vi "GetCOMPortold.vi"(8 "error in (no error)":errorcluster caption="错误输入（无错误）") -> (0 "error out":errorcluster caption="错误输出", 2 "COMPort":refnum<visa-resource-name>[](array[refnum]))   [LabVIEW 2013]
uses:
  <vilib>/nisyscfg/Filter Mode.ctl
  <vilib>/nisyscfg/Close (System).vi
  <vilib>/nisyscfg/nisyscfg.lvlib
  <resource>/objmgr/nisysapi.rc
panel:
  out "数组":string[](array[string])
  out "Alias":string[](array[string])
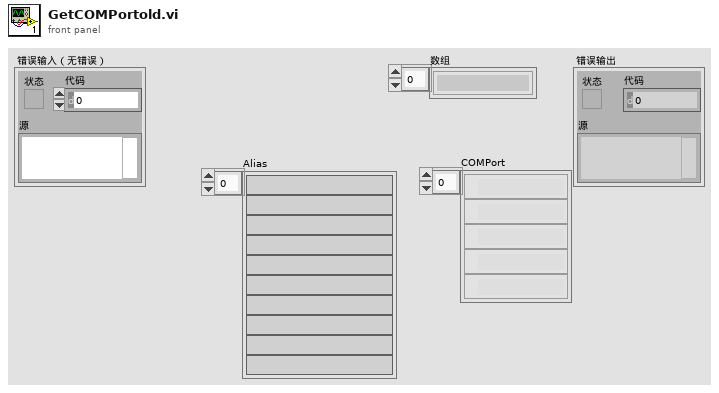
[diagram p1: front panel]
types:
  T1 = typedef "nisyscfg.lvlib/Filter Mode.ctl" = i32
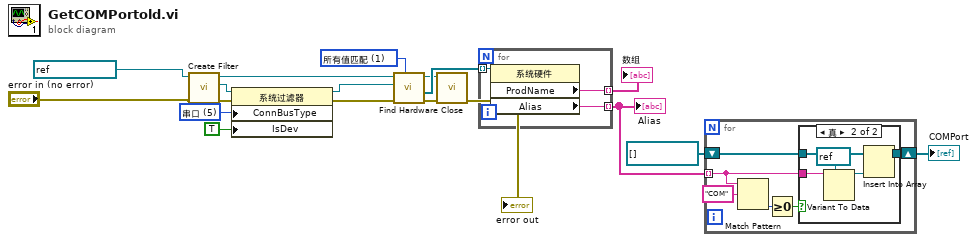
[diagram p0: block diagram]
diagram:
  w14 = u32 5 items=["内置/系统", "PXI/PCI", "USB", "GPIB", "VXI", "串口", "TCP/IP", "cRIO", "SCXI", "cDAQ", "SwitchBlock", "SCC", "FireWire", "FlexAdapter", "CAN"] ("设备与机箱:提供总线类型")
  w17 = T1 1 items=["所有值匹配"=1, "任意值匹配"=2, "值不匹配"=3, "所有属性存在"=4] ("Filter Mode (all values match)")
  n1 = call <vilib>:"Create Filter.vi"("error in (no error)"="error in (no error)", "Session in"=refnum<k21> "localhost") -> ("error out"=w16:errorcluster, "Filter out"=w10:refnum<k20>, "Session out"=w12:refnum<k21>)  [unwired: 7 in]
  n2 = property class="系统过滤器"(reference=w10, error in=w16, "ConnBusType"=w14, "IsDev"=TRUE ("属于设备")) -> (reference out=w9:refnum<k20>, error out=w11:errorcluster)
  n3 = call <vilib>:"Find Hardware.vi"("Filter Mode (all values match)"=w17, "error in (no error)"=w11, "Filter in"=w9, "Session in"=w12) -> ("error out"=w13:errorcluster, "Resources out"=w18:refnum<k20>[], "Session out"=w15:refnum<k21>)  [unwired: 4 in, 1 out]
  n4 = call-poly <vilib>:"Close.vi"("error in (no error)"=w13, "Session in"=w15) -> ("error out"=→"error out":errorcluster)  [unwired: 9 in]
  n5 = for {
    tunnel: w18 -> [w21] mode=indexing
    tunnel: [w20] -> w3 mode=indexing
    tunnel: [w19] -> w7 mode=indexing
    n6 = property class="系统硬件"(reference=w21) -> ("ProdName"=w20:string, "Alias"=w19:string)  [unwired: 1 in, 2 out]
  }
  "Alias" <- w7
  "数组" <- w3
  n7 = for {
    tunnel: w7 -> [w24] mode=indexing
    shift-right: [w23] -> w5
    shift-left: refnum<visa-resource-name>[] [] -> [w22]
    n8 = Match Pattern(string=w24, regular expression="COM" ("正则表达式")) -> (offset past match=w26:i32)  [unwired: 1 in, 3 out]
    n9 = Greater Or Equal To 0?(x=w26) -> (x >= 0?=w25:bool)
    n10 = case shown="真" w25 {
      tunnel: w24 -> [_ w32]
      tunnel: [w28 w30] -> w23
      tunnel: w22 -> [w28 w29]
      frame False {
      }
      frame True {
        n11 = Variant To Data(type=refnum<visa-resource-name> refnum ("VISA resource name"), Variant=w32) -> (data=w31:refnum<visa-resource-name>)  [unwired: 1 in, 1 out]
        n12 = Insert Into Array(array=w29, new element=w31) -> (w30:refnum<visa-resource-name>[])  [unwired: 1 in]
      }
    }
  }
  "COMPort" <- w5
